vi "Get Internal Command FIFO References.vi"(8 "error in (no error)":errorcluster, 11 "Internal Command Engine References":T1 {"Response Refs"."Block Data Refs" format="%.0x"; "Command Refs"."Block Data Refs"."Data Reference" format="%.0x"}) -> (0 "error out":errorcluster, 3 "Internal Command Engine References":T4 {"Command Refs"."Block Data Refs"."Data Reference" format="%.0x"; "Response Refs"."Block Data Refs" format="%.0x"})   [LabVIEW 2013, in "J1939 Addon Engine.lvlib"]
uses:
  J1939 Addon Engine.lvlib
  Types/Internal Command Configuration Parameters.ctl
  <vilib>/NI Veristand/Custom Device API/Data Reference.ctl
  <vilib>/NI Veristand/Custom Device API/Block Data Reference.ctl
  Shared/Types/SysDef Command Settings.ctl
  <vilib>/NI Veristand/Custom Device API/Custom Device API.lvlib
  Shared/J1939 Addon Shared.lvlib
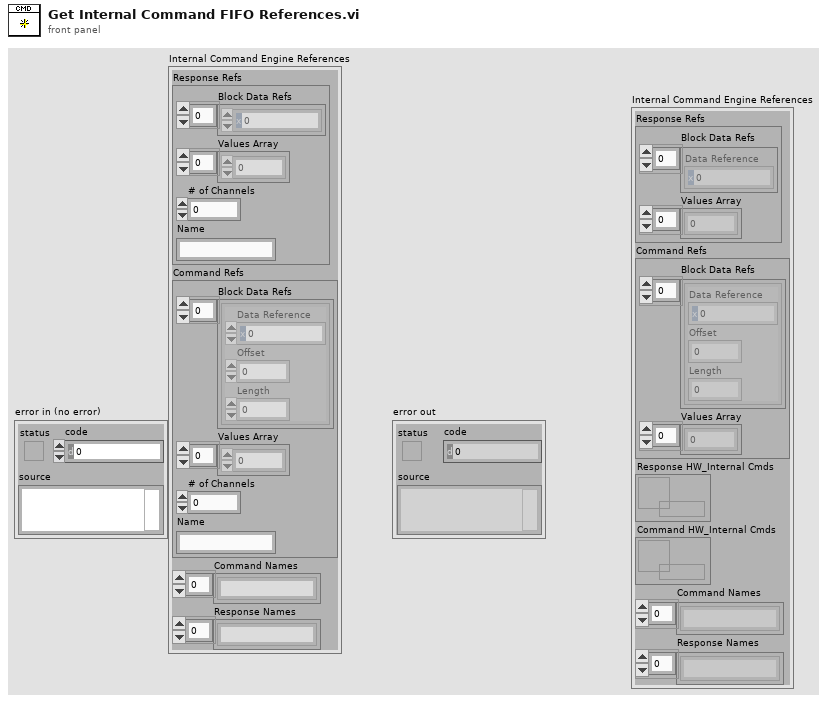
[diagram p1: front panel]
types:
  T1 = typedef "J1939 Addon Shared.lvlib/SysDef Command Settings.ctl" = cluster{"Response Refs":cluster{"Block Data Refs":T2[], "Values Array":dbl[], "# of Channels":u32, "Name":string}, "Command Refs":cluster{"Block Data Refs":T3[], "Values Array":dbl[], "# of Channels":u32, "Name":string}, "Command Names":string[], "Response Names":string[]}
  T2 = typedef "Custom Device API.lvlib/Data Reference.ctl" = i32
  T3 = typedef "Custom Device API.lvlib/Block Data Reference.ctl" = cluster{"Data Reference":T2, "Offset":i32, "Length":i32}
  T4 = typedef "J1939 Addon Engine.lvlib/Internal Command Configuration Parameters.ctl" = cluster{"Response Refs":cluster{"Block Data Refs":T2[], "Values Array":dbl[]}, "Command Refs":cluster{"Block Data Refs":T3[], "Values Array":dbl[]}, "Response HW_Internal Cmds":refnum<k33>, "Command HW_Internal Cmds":refnum<k33>, "Command Names":string[], "Response Names":string[]}
  T5 = cluster{"read mode":enum16{"polling", "blocking"}, "write mode":enum16{"polling", "blocking"}}
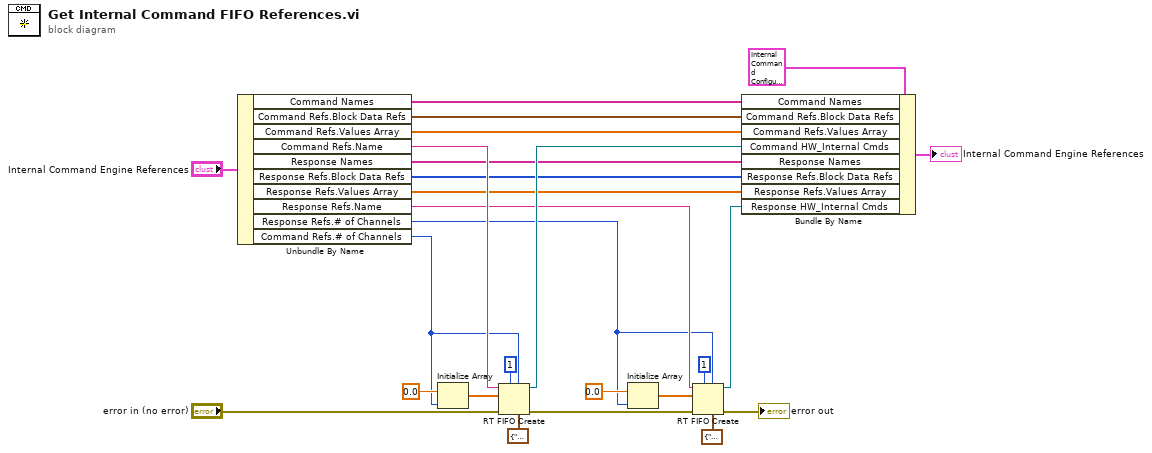
[diagram p0: block diagram]
diagram:
  n1 = Unbundle By Name("Internal Command Engine References") -> ("Command Names"=w13:string[], "Command Refs.Block Data Refs"=w12:T3[], "Command Refs.Values Array"=w11:dbl[], "Command Refs.Name"=w10:string, "Response Names"=w8:string[], "Response Refs.Block Data Refs"=w7:T2[], "Response Refs.Values Array"=w6:dbl[], "Response Refs.Name"=w4:string, "Response Refs.# of Channels"=w2:u32, "Command Refs.# of Channels"=w1:u32)
  n2 = Initialize Array(0.0 ("element"), w1) -> (w26:dbl[])
  n3 = RT FIFO Create(0:w10, 1:w26, 3:"error in (no error)", 4:u32 1 ("size (10)"), 6:w1, 7:T5 {"read mode"=enum."blocking", "write mode"=enum."polling"} ("r/w modes (polling,polling)")) -> (8:w17:refnum<k33>, 11:w3:errorcluster)  [unwired: 2 in, 1 out]
  n4 = Initialize Array(0.0 ("element"), w2) -> (w5:dbl[])
  n5 = RT FIFO Create(0:w4, 1:w5, 3:w3, 4:u32 1 ("size (10)"), 6:w2, 7:T5 {"read mode"=enum."blocking", "write mode"=enum."polling"} ("r/w modes (polling,polling)")) -> (8:w16:refnum<k33>, 11:→"error out":errorcluster)  [unwired: 2 in, 1 out]
  n6 = Bundle By Name(cluster=T4 {"Response Refs"={"Block Data Refs"=[], "Values Array"=[]}, "Command Refs"={"Block Data Refs"=[], "Values Array"=[]}, "Response HW_Internal Cmds"=refnum, "Command HW_Internal Cmds"=refnum, "Command Names"=[], "Response Names"=[]} ("Internal Command Engine References"), "Command Names"=w13, "Command Refs.Block Data Refs"=w12, "Command Refs.Values Array"=w11, "Command HW_Internal Cmds"=w17, "Response Names"=w8, "Response Refs.Block Data Refs"=w7, "Response Refs.Values Array"=w6, "Response HW_Internal Cmds"=w16) -> (→"Internal Command Engine References":T4)
